vi "Signal Processing subVI.vi"(0 "data":waveform(dbl), 5 "Bass":dbl, 7 "Mid-tone":dbl, 9 "Treble":dbl, 11 "error in (no error)":errorcluster) -> (4 "Power Spectrum / PSD":cluster{"f0":dbl, "df":dbl, "magnitude":dbl[]}, 8 "output waveform":waveform(dbl), 15 "error out":errorcluster)   [LabVIEW 2013]
uses:
  <vilib>/measure/macond.llb/IIR Filter for 1 Chan.vi
  <vilib>/measure/maspectr.llb/FFT Power Spectrum and PSD for 1 Chan.vi
  <vilib>/measure/NI_MAPro.lvlib
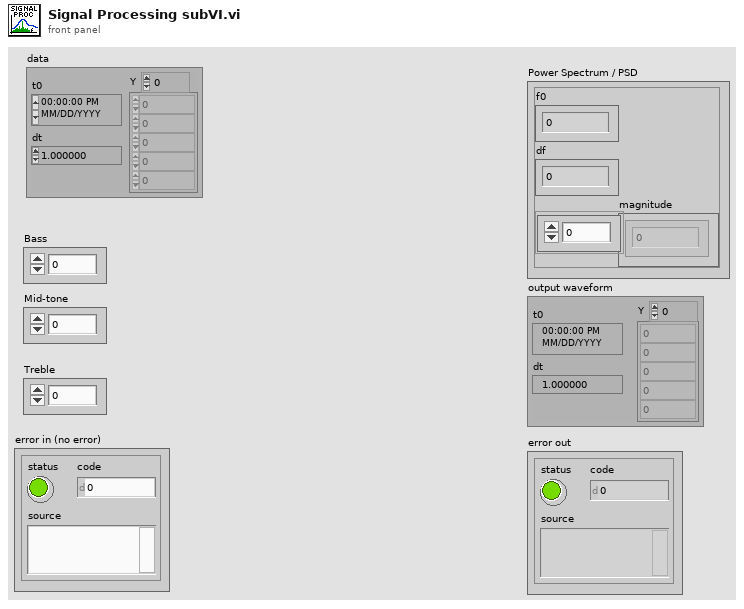
[diagram p1: front panel]
types:
  T1 = cluster{"Topology":enum16{"Off", "Butterworth", "Chebyshev", "Inverse Chebyshev", "Elliptic", "Bessel"}, "Type":enum16{"Lowpass", "Highpass", "Bandpass", "Bandstop"}, "Order":i32, "Lower Fc":dbl, "Upper Fc":dbl, "PB Ripple":dbl, "SB Attenuation":dbl}
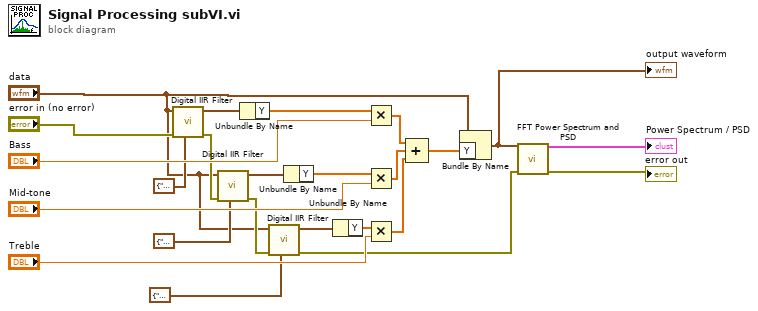
[diagram p0: block diagram]
diagram:
  n1 = call-poly <vilib>:"Digital IIR Filter.vi"("IIR filter specifications"=T1 {"Topology"=enum."Butterworth", "Type"=enum."Lowpass", "Order"=10, "Lower Fc"=600.0, "Upper Fc"=200.0, "PB Ripple"=1.0, "SB Attenuation"=60.0}, "error in (no error)"="error in (no error)", "signal in"="data") -> ("error out"=w8:errorcluster, "signal out"=w23:waveform(dbl))  [unwired: 6 in, 1 out]
  n2 = call-poly <vilib>:"Digital IIR Filter.vi"("IIR filter specifications"=T1 {"Topology"=enum."Butterworth", "Type"=enum."Bandpass", "Order"=10, "Lower Fc"=800.0, "Upper Fc"=4000.0, "PB Ripple"=1.0, "SB Attenuation"=60.0}, "error in (no error)"=w8, "signal in"="data") -> ("error out"=w9:errorcluster, "signal out"=w11:waveform(dbl))  [unwired: 6 in, 1 out]
  n3 = Unbundle By Name(w23) -> ("Y"=w13:dbl[])
  n4 = call-poly <vilib>:"Digital IIR Filter.vi"("IIR filter specifications"=T1 {"Topology"=enum."Butterworth", "Type"=enum."Highpass", "Order"=10, "Lower Fc"=5000.0, "Upper Fc"=200.0, "PB Ripple"=1.0, "SB Attenuation"=60.0}, "error in (no error)"=w9, "signal in"="data") -> ("error out"=w10:errorcluster, "signal out"=w12:waveform(dbl))  [unwired: 6 in, 1 out]
  n5 = Unbundle By Name(w11) -> ("Y"=w14:dbl[])
  n6 = Unbundle By Name(w12) -> ("Y"=w15:dbl[])
  n7 = Multiply(x=w13, y="Bass") -> (x*y=w19:dbl[])
  n8 = Multiply(x=w14, y="Mid-tone") -> (x*y=w21:dbl[])
  n9 = Multiply(x=w15, y="Treble") -> (x*y=w20:dbl[])
  n10 = Compound Arithmetic op=ADD(w19, w21, w20) -> (w22:dbl[])
  n11 = Bundle By Name(cluster="data", "Y"=w22) -> (w24:waveform(dbl))
  "output waveform" <- w24
  n12 = call-poly <vilib>:"FFT Power Spectrum and PSD.vi"("error in (no error)"=w10, "time signal"=w24) -> ("error out"=→"error out":errorcluster, "Power Spectrum / PSD"=→"Power Spectrum / PSD":cluster{"f0":dbl, "df":dbl, "magnitude":dbl[]})  [unwired: 6 in, 2 out]
